vi "HexToFloat.vi"(11 "数组输入":u16[](array[numeric]) format="%xH") -> (3 "数组输出":sgl[](array[numeric]))   [LabVIEW 2016, in "超标留样集成.lvlib" / "ESTD1200.lvlib"]
uses:
  ESTD1200.lvlib
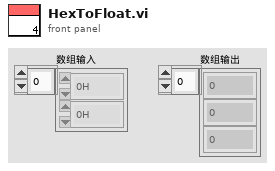
[diagram p1: front panel]
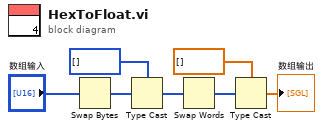
[diagram p0: block diagram]
diagram:
  n1 = Swap Bytes(anything="数组输入") -> (byte swapped=w5:u16[])
  n2 = Type Cast(type=u32[] [], x=w5) -> (*(type *) &x=w3:u32[])
  n3 = Swap Words(1:w3) -> (0:w4:u32[])
  n4 = Type Cast(type=sgl[] [], x=w4) -> (*(type *) &x=→"数组输出":sgl[])
